vi "ProcessData.vi"(8 "error in (no error)":errorcluster, 9 "State":T1, 10 "Analog Data":T3, 11 "WhiteNoiseOrientationDetection in":refnum<class "WhiteNoiseOrientationDetection.lvclass">) -> (0 "error out":errorcluster, 1 "Fixated":bool, 2 "Trigger":T2=enum."Broke Fixation", 3 "WhiteNoiseOrientationDetection out":refnum<class "WhiteNoiseOrientationDetection.lvclass">)   [LabVIEW 2012, in "WhiteNoiseOrientationDetection.lvclass"]
uses:
  WhiteNoiseOrientationDetection.lvclass
  Core SubVIs/Controls/TYPE - Analog Data.ctl
  Trial Based Experiment Statechart/Trial Based Experiment.lvsc/Trigger.ctl
  Trial Based Experiment Statechart/Trial Based Experiment.lvsc/State.ctl
  WhiteNoiseOrientationDetection.lvclass/WhiteNoiseOrientationDetection.ctl
  <vilib>/measure/madcrms.llb/Basic Averaged DC-RMS for 1 Chan.vi
  Trial Based Experiment Statechart/Trial Based Experiment.lvsc
  Core SubVIs/Core SubVIs.lvlib
  <vilib>/measure/NI_MAPro.lvlib
  Acquisition/BehaviorData/BehaviorData.lvclass
panel:
  out "Response Window":bool
  in  "Adjustment Rate":dbl=0.02
  in  "Toggle Fixation":bool
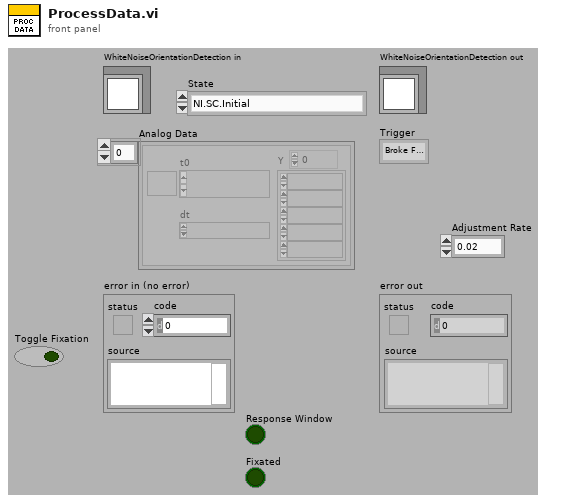
[diagram p1: front panel]
types:
  T1 = typedef "Trial Based Experiment.lvsc/State.ctl" = enum16{"NI.SC.Initial", "NI.SC.History", "NI.SC.ShallowHistory", "NI.SC.Terminal", "Cleanup", "State", "State\\Region\\Pause", "State\\Region\\Response Period", "State\\Region\\Delay Period", "State\\Region\\Hold Fixation", "State\\Region\\Acquire Fixation", "State\\Region\\Abort Trial", "State\\Region\\End Trial", "State\\Region\\Intertrial", "State\\Region\\Start Trial"}
  T2 = typedef "Trial Based Experiment.lvsc/Trigger.ctl" = enum16{"NULL", "Fixated", "Broke Fixation", "Stop", "Correct Response", "Incorrect Response", "Timeout"}
  T3 = typedef "Core SubVIs.lvlib/TYPE - Analog Data.ctl" = waveform(dbl)[]
  T4 = enum16{"Get Time", "Get Elapsed Time", "Reset Elapsed Time"}
  T5 = cluster{"Intertrial":dbl, "AcquireFixation":dbl, "HoldFixation":dbl, "DelayPeriod":dbl, "ResponsePeriod":dbl}
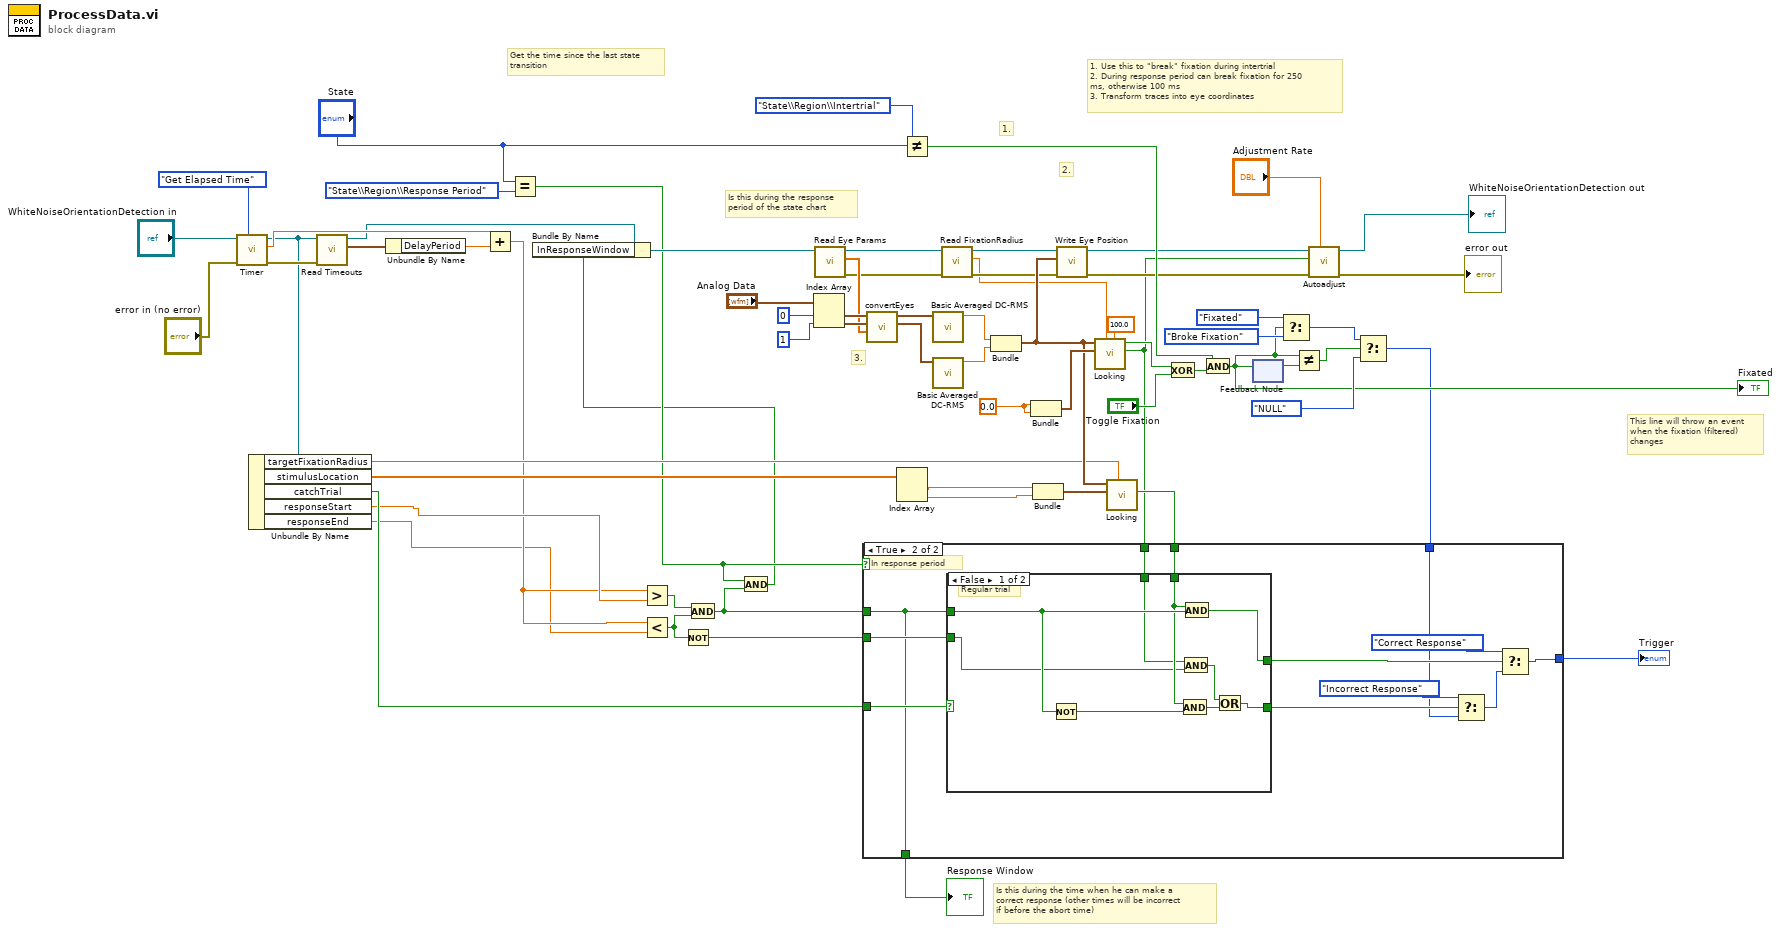
[diagram p0: block diagram]
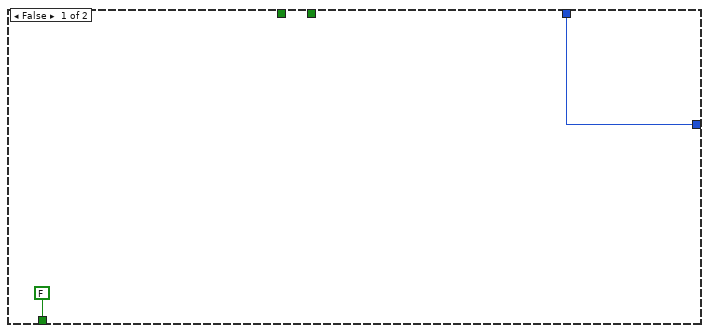
[diagram p2: hidden frame]
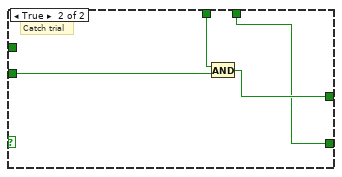
[diagram p3: hidden frame]
diagram:
  w53 = 0.0
  # "Is this during the time when he can make a\ncorrect response (other times will be incorrect\nif before the abort time)"
  # "Is this during the response\nperiod of the state chart"
  # "Get the time since the last state\ntransition"
  # "This line will throw an event\nwhen the fixation (filtered)\nchanges"
  # "3."
  # "1."
  # "2."
  # "1. Use this to \"break\" fixation during intertrial\n2. During response period can break fixation for 250\nms, otherwise 100 ms\n3. Transform traces into eye coordinates"
  n1 = call-dynamic "Timer.vi"("Method"=T4."Get Elapsed Time", "error in (no error)"="error in (no error)", "BehaviorData in"="WhiteNoiseOrientationDetection in") -> ("error out"=w31:errorcluster, "Time"=w28:dbl, "BehaviorData out"=w23:refnum<class "WhiteNoiseOrientationDetection.lvclass">)  [unwired: 5 in, 1 out]
  n2 = Unbundle By Name(w23) -> ("targetFixationRadius"=w19:dbl, "stimulusLocation"=w22:dbl[], "catchTrial"=w13:bool, "responseStart"=w10:dbl, "responseEnd"=w8:dbl)
  n3 = call-dynamic "Read Timeouts.vi"("error in (no error)"=w31, "TrialBasedExperiment in"=w23) -> ("Timeouts"=w30:T5, "TrialBasedExperiment out"=w18:refnum<class "WhiteNoiseOrientationDetection.lvclass">)  [unwired: 7 in, 1 out]
  n4 = Unbundle By Name(w30) -> ("DelayPeriod"=w29:dbl)
  n5 = Add(x=w28, y=w29) -> (x+y=w9:dbl)
  n6 = Equal?(x="State", y=State."State\\Region\\Response Period") -> (x = y?=w5:bool)
  n7 = Greater?(x=w9, y=w10) -> (0:w11:bool)
  n8 = Less?(x=w9, y=w8) -> (x < y?=w12:bool)
  n9 = Not(x=w12) -> (.not. x?=w7:bool)
  n10 = And(x=w11, y=w12) -> (x .and. y?=w4:bool)
  n11 = And(x=w5, y=w4) -> (x .and. y?=w3:bool)
  n12 = Bundle By Name(cluster=w18, "InResponseWindow"=w3) -> (w17:refnum<class "WhiteNoiseOrientationDetection.lvclass">)
  n13 = Index Array(array="Analog Data", index #1=0 ("index"), index #2=1 ("index")) -> (element #1=w67:waveform(dbl), element #2=w66:waveform(dbl))
  n14 = call-dynamic "Read Eye Params.vi"("TrialBasedExperiment in"=w17) -> ("error out"=w48:errorcluster, "Eye Params"=w58:dbl[], "TrialBasedExperiment out"=w27:refnum<class "WhiteNoiseOrientationDetection.lvclass">)  [unwired: 8 in]
  n15 = call "convertEyes.vi"("Params"=w58, "Vertical"=w66, "Horizontal"=w67) -> ("Vertical Calibrated"=w64:waveform(dbl), "Horizontal Calibrated"=w65:waveform(dbl))  [unwired: 7 in]
  n16 = Index Array(array=w22) -> (element #1=w21:dbl, element #2=w20:dbl)  [unwired: 2 in]
  n17 = Not Equal?(x=State."State\\Region\\Intertrial", y="State") -> (x != y?=w42:bool)
  n18 = call-poly <vilib>:"Basic Averaged DC-RMS.vi"("signal in"=w65) -> ("DC value"=w56:dbl)  [unwired: 7 in, 3 out]
  n19 = call-poly <vilib>:"Basic Averaged DC-RMS.vi"("signal in"=w64) -> ("DC value"=w55:dbl)  [unwired: 7 in, 3 out]
  n20 = call-dynamic "Read FixationRadius.vi"("error in (no error)"=w48, "MatlabExperiment in"=w27) -> ("error out"=w46:errorcluster, "FixationRadius"=w45:dbl, "MatlabExperiment out"=w47:refnum<class "WhiteNoiseOrientationDetection.lvclass">)  [unwired: 7 in]
  n21 = Bundle("DC value"=w56, "DC value"=w55) -> (w49:cluster{"DC value":dbl, "DC value":dbl})  [unwired: 1 in]
  n22 = Bundle(w53, w53) -> (w54:cluster{dbl, dbl})  [unwired: 1 in]
  n23 = Bundle("Numeric"=w21, "Numeric"=w20) -> (w50:cluster{"Numeric":dbl, "Numeric":dbl})  [unwired: 1 in]
  n24 = call-dynamic "Write Eye Position.vi"("error in (no error)"=w46, "Eye Position"=w49, "TrialBasedExperiment in"=w47) -> ("error out"=w38:errorcluster, "TrialBasedExperiment out"=w39:refnum<class "WhiteNoiseOrientationDetection.lvclass">)  [unwired: 7 in]
  n25 = call "Looking.vi"("Break Timeout (ms)"=100.0 ("f"), "Fixation Radius (px)"=w45, "Desired Position"=w54, "Eye Position"=w49) -> ("Looking Unfiltered"=w14:bool, "Looking"=w51:bool)  [unwired: 6 in]
  n26 = call "Looking.vi"("Fixation Radius (px)"=w19, "Desired Position"=w50, "Eye Position"=w49) -> ("Looking Unfiltered"=w15:bool)  [unwired: 7 in, 1 out]
  n27 = Exclusive Or(1:"Toggle Fixation", 2:w51) -> (0:w43:bool)
  n28 = And(x=w42, y=w43) -> (x .and. y?=w25:bool)
  "Fixated" <- w25
  n29 = feedback #1() -> (w63:bool)  [unwired: 1 in]
  n30 = feedback-in #1(w25) -> ()
  n31 = Select(t=Trigger."Fixated" ("Trigger"), s=w25, f=Trigger."Broke Fixation" ("Trigger")) -> (s? t:f=w61:T2)
  n32 = Not Equal?(x=w25, y=w63) -> (x != y?=w40:bool)
  n33 = call-dynamic "Autoadjust.vi"("Adjustment Rate"="Adjustment Rate", "error in (no error)"=w38, "Fixated"=w14, "TrialBasedExperiment in"=w39) -> ("error out"=→"error out":errorcluster, "TrialBasedExperiment out"=→"WhiteNoiseOrientationDetection out":refnum<class "WhiteNoiseOrientationDetection.lvclass">)  [unwired: 6 in]
  n34 = Select(t=w61, s=w40, f=Trigger."NULL" ("Trigger")) -> (s? t:f=w2:T2)
  n35 = case shown="True" w5 {
    tunnel: w15 -> [_ w77]
    tunnel: [w69 w81] -> w1
    tunnel: w14 -> [_ w79]
    tunnel: w13 -> [_ w80]
    tunnel: w4 -> [_ w75]
    tunnel: w7 -> [_ w76]
    tunnel: [FALSE w75] -> w6
    tunnel: w2 -> [w69 w71]
    frame False {
    }
    frame True {
      # "In response period"
      n36 = case shown="False" w80 {
        tunnel: w79 -> [w87 w95]
        tunnel: [w91 w94] -> w78
        tunnel: w77 -> [w89 w92]
        tunnel: w75 -> [w90 _]
        tunnel: w76 -> [w86 w93]
        tunnel: [w83 w92] -> w72
        frame False {
          # "Regular trial"
          n37 = Not(x=w90) -> (.not. x?=w88:bool)
          n38 = And(x=w89, y=w88) -> (x .and. y?=w85:bool)
          n39 = And(x=w87, y=w86) -> (x .and. y?=w84:bool)
          n40 = And(x=w89, y=w90) -> (x .and. y?=w91:bool)
          n41 = Or(x=w84, y=w85) -> (x .or. y?=w83:bool)
        }
        frame True {
          # "Catch trial"
          n42 = And(x=w95, y=w93) -> (x .and. y?=w94:bool)
        }
      }
      n43 = Select(t=Trigger."Incorrect Response", s=w72, f=w71) -> (s? t:f=w73:T2)
      n44 = Select(t=Trigger."Correct Response", s=w78, f=w73) -> (s? t:f=w81:T2)
    }
  }
  "Trigger" <- w1
  "Response Window" <- w6
